vi "InitArray.vi"(8 "Index":i32, 11 "Array In":dbl[](array[numeric])) -> (3 "Array Out":dbl[](array[numeric]))   [LabVIEW 2017]
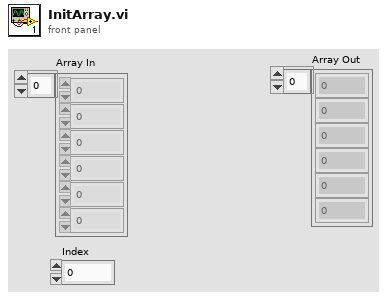
[diagram p1: front panel]
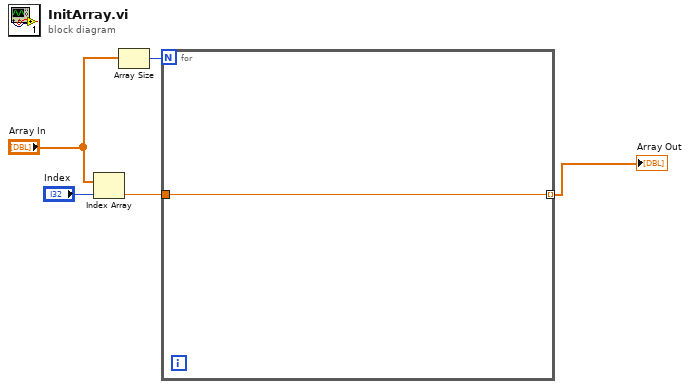
[diagram p0: block diagram]
diagram:
  n1 = Index Array(array="Array In", index="Index") -> (element=w2:dbl)
  n2 = Array Size(array="Array In") -> (size(s)=w4:i32)
  n3 = for {
    N: w4 -> [_]
    tunnel: w2 -> [w6]
    tunnel: [w6] -> w1 mode=indexing
  }
  "Array Out" <- w1
